vi "GlobalDrivebase.vi"() -> ()   [LabVIEW 2023]
panel:
  in  "DriveConfig":T1={"Future Proof Configs"=FALSE, "MotorOutputInverted"=0, "MotorOutputNeutralMode"=0, "MotorOutputDutyCycleNeutralDeadband"=0.0, "MotorOutputPeakForwardDutyCycle"=1.0, "MotorOutputPeakReverseDutyCycle"=-1.0, "CurrentLimitsStatorCurrentLimit"=0.0, "CurrentLimitsStatorCurrentLimitEnable"=FALSE, "CurrentLimitsSupplyCurrentLimit"=0.0, "CurrentLimitsSupplyCurrentLimitEnable"=FALSE, "CurrentLimitsSupplyCurrentThreshold"=0.0, "CurrentLimitsSupplyTimeThreshold"=0.0, "VoltageSupplyVoltageTimeConstant"=0.0, "VoltagePeakForwardVoltage"=16.0, "VoltagePeakReverseVoltage"=-16.0, "TorqueCurrentPeakForwardTorqueCurrent"=800.0, "TorqueCurrentPeakReverseTorqueCurrent"=-800.0, "TorqueCurrentTorqueNeutralDeadband"=0.0, "FeedbackFeedbackRotorOffset"=0.0, "FeedbackSensorToMechanismRatio"=1.0, "FeedbackRotorToSensorRatio"=1.0, "FeedbackFeedbackSensorSource"=0, "FeedbackFeedbackRemoteSensorID"=0, "DifferentialSensorsDifferentialSensorSource"=0, "DifferentialSensorsDifferentialTalonFXSensorID"=0, "DifferentialSensorsDifferentialRemoteSensorID"=0, "DifferentialConstantsPeakDifferentialDutyCycle"=2.0, "DifferentialConstantsPeakDifferentialVoltage"=32.0, "DifferentialConstantsPeakDifferentialTorqueCurrent"=1600.0, "OpenLoopRampsDutyCycleOpenLoopRampPeriod"=0.0, "OpenLoopRampsVoltageOpenLoopRampPeriod"=0.0, "OpenLoopRampsTorqueOpenLoopRampPeriod"=0.0, "ClosedLoopRampsDutyCycleClosedLoopRampPeriod"=0.0, "ClosedLoopRampsVoltageClosedLoopRampPeriod"=0.0, "ClosedLoopRampsTorqueClosedLoopRampPeriod"=0.0, "HardwareLimitSwitchForwardLimitType"=0, "HardwareLimitSwitchForwardLimitAutosetPositionEnable"=FALSE, "HardwareLimitSwitchForwardLimitAutosetPositionValue"=0.0, "HardwareLimitSwitchForwardLimitEnable"=TRUE, "HardwareLimitSwitchForwardLimitSource"=0, "HardwareLimitSwitchForwardLimitRemoteSensorID"=0, "HardwareLimitSwitchReverseLimitType"=0, "HardwareLimitSwitchReverseLimitAutosetPositionEnable"=FALSE, "HardwareLimitSwitchReverseLimitAutosetPositionValue"=0.0, "HardwareLimitSwitchReverseLimitEnable"=TRUE, "HardwareLimitSwitchReverseLimitSource"=0, "HardwareLimitSwitchReverseLimitRemoteSensorID"=0, "AudioBeepOnBoot"=TRUE, "AudioBeepOnConfig"=TRUE, "AudioAllowMusicDurDisable"=FALSE, "SoftwareLimitSwitchForwardSoftLimitEnable"=FALSE, "SoftwareLimitSwitchReverseSoftLimitEnable"=FALSE, "SoftwareLimitSwitchForwardSoftLimitThreshold"=0.0, "SoftwareLimitSwitchReverseSoftLimitThreshold"=0.0, "MotionMagicMotionMagicCruiseVelocity"=0.0, "MotionMagicMotionMagicAcceleration"=0.0, "MotionMagicMotionMagicJerk"=0.0, "MotionMagicMotionMagicExpo_kV"=0.0, "MotionMagicMotionMagicExpo_kA"=0.0, "CustomParamsCustomParam0"=0, "CustomParamsCustomParam1"=0, "ClosedLoopGeneralContinuousWrap"=FALSE, "Slot0kP"=0.0, "Slot0kI"=0.0, "Slot0kD"=0.0, "Slot0kS"=0.0, "Slot0kV"=0.0, "Slot0kA"=0.0, "Slot0kG"=0.0, "Slot0GravityType"=0, "Slot0StaticFeedforwardSign"=0, "Slot1kP"=0.0, "Slot1kI"=0.0, "Slot1kD"=0.0, "Slot1kS"=0.0, "Slot1kV"=0.0, "Slot1kA"=0.0, "Slot1kG"=0.0, "Slot1GravityType"=0, "Slot1StaticFeedforwardSign"=0, "Slot2kP"=0.0, "Slot2kI"=0.0, "Slot2kD"=0.0, "Slot2kS"=0.0, "Slot2kV"=0.0, "Slot2kA"=0.0, "Slot2kG"=0.0, "Slot2GravityType"=0, "Slot2StaticFeedforwardSign"=0} {"MotorOutputInverted" items=["CounterClockwise_Positive", "Clockwise_Positive"]; "MotorOutputNeutralMode" items=["Coast", "Brake"]; "FeedbackFeedbackSensorSource" items=["RotorSensor", "RemoteCANcoder", "RemotePigeon2_Yaw", "RemotePigeon2_Pitch", "RemotePigeon2_Roll", "FusedCANcoder", "SyncCANcoder"]; "DifferentialSensorsDifferentialSensorSource" items=["Disabled", "RemoteTalonFX_Diff", "RemotePigeon2_Yaw", "RemotePigeon2_Pitch", "RemotePigeon2_Roll", "RemoteCANcoder"]; "HardwareLimitSwitchForwardLimitType" items=["NormallyOpen", "NormallyClosed"]; "HardwareLimitSwitchForwardLimitSource" items=["LimitSwitchPin"=0, "RemoteTalonFX"=1, "RemoteCANifier"=2, "RemoteCANcoder"=4, "Disabled"=3]; "HardwareLimitSwitchReverseLimitType" items=["NormallyOpen", "NormallyClosed"]; "HardwareLimitSwitchReverseLimitSource" items=["LimitSwitchPin"=0, "RemoteTalonFX"=1, "RemoteCANifier"=2, "RemoteCANcoder"=4, "Disabled"=3]; "Slot0GravityType" items=["Elevator_Static", "Arm_Cosine"]; "Slot0StaticFeedforwardSign" items=["UseVelocitySign", "UseClosedLoopSign"]; "Slot1GravityType" items=["Elevator_Static", "Arm_Cosine"]; "Slot1StaticFeedforwardSign" items=["UseVelocitySign", "UseClosedLoopSign"]; "Slot2GravityType" items=["Elevator_Static", "Arm_Cosine"]; "Slot2StaticFeedforwardSign" items=["UseVelocitySign", "UseClosedLoopSign"]}
  out "SEN_Shifter_Stuck":bool[](array[boolean])
  out "SEN_Shifter_Failure":bool[](array[boolean])
  in  "SEN_Actual_Shifter_State_3":T2(ring)
  in  "SEN_Actual_Shifter_State_2":T2(ring)
  in  "SEN_Actual_Shifter_State_1":T2(ring)
  in  "SEN_Actual_Shifter_State_0":T2(ring)
  out "OUT_Heading_Locked":bool
  out "CON_Nominal_Drive_Wheel_Diameter (in)":dbl
  out "OUT_Auto-Targeting":bool
  out "SEN_Drive_Fault":bool[](array[boolean])
  out "DAT_Unlock_Azimuth":bool
  out "OUT_Azimuth_Error_3 (deg)":dbl
  out "OUT_Azimuth_Error_1 (deg)":dbl
  out "OUT_Azimuth_Error_2 (deg)":dbl
  out "OUT_Azimuth_Error_0 (deg)":dbl
  out "SEN_Drive_Raw_Velocity_2 (rpm)":dbl
  out "SEN_Drive_Raw_Velocity_3 (rpm)":dbl
  out "SEN_Drive_Raw_Velocity_1 (rpm)":dbl
  out "SEN_Drive_Raw_Velocity_0 (rpm)":dbl
  out "DAT_Auto_Targeting_Override":bool
  out "SEN_Azimuth_Position_Unwrapped_3 (deg)":dbl
  out "SEN_Azimuth_Position_Unwrapped_2 (deg)":dbl
  out "SEN_Azimuth_Position_Unwrapped_1 (deg)":dbl
  out "SEN_Azimuth_Position_Unwrapped_0 (deg)":dbl
  out "SEN_Latched_Shift_Time_3 (ms)":u32
  out "SEN_Latched_Shift_Time_2 (ms)":u32
  out "SEN_Latched_Shift_Time_1 (ms)":u32
  out "SEN_Latched_Shift_Time_0 (ms)":u32
  out "SEN_Drive_Velocity_2 (ft/s)":dbl
  out "SEN_Drive_Velocity_3 (ft/s)":dbl
  out "SEN_Drive_Velocity_1 (ft/s)":dbl
  out "SEN_Drive_Velocity_0 (ft/s)":dbl
  out "SEN_Drive_Overheat":bool[](array[boolean])
  out "SEN_Azimuth_Fault":bool[](array[boolean])
  out "SEN_Drive_Temp_2 (C)":dbl
  out "SEN_Drive_Temp_3 (C)":dbl
  out "SEN_Drive_Temp_1 (C)":dbl
  out "SEN_Drive_Temp_0 (C)":dbl
  out "SEN_Azimuth_Position_3 (deg)":dbl
  out "SEN_Azimuth_Position_2 (deg)":dbl
  out "SEN_Azimuth_Position_1 (deg)":dbl
  out "SEN_Azimuth_Position_0 (deg)":dbl
  out "OUT_Orientation Mode":enum16{"Robot-Oriented", "Field-Oriented"}(ring)
  out "OUT_Current_Driver_Profile_Setpoints":dbl[](array[numeric])
  out "OUT_Force_Low_Gear":bool
  out "OUT_High_Gear_Requested_2":bool
  out "OUT_High_Gear_Requested_1":bool
  out "OUT_High_Gear_Requested_3":bool
  out "OUT_High_Gear_Requested_0":bool
  out "OUT_Azimuth_Goal_3 (deg)":dbl
  out "OUT_Azimuth_Goal_1 (deg)":dbl
  out "OUT_Azimuth_Goal_2 (deg)":dbl
  out "OUT_Azimuth_Goal_0 (deg)":dbl
  out "OUT_Swerve_Rotation_Command":dbl
  out "OUT_Boost_Drive_Train":bool
  out "OUT_Drive_Command_3":dbl
  out "OUT_Drive_Command_1":dbl
  out "OUT_Drive_Command_2":dbl
  out "OUT_Drive_Command_0":dbl
  out "CON_Legal_Drivers":string[](array[string])
  out "DAT_New_Driver_Profile_Setpoints":dbl[](array[numeric])
  out "DAT_Apply_Driver_Profile_Setpoints":bool
  out "DAT_Starting_IMU_Reset":bool
  out "DAT_Field_Oriented_Override":bool
  out "DAT_Home_Wheels":bool
  out "DAT_Calibrate_Wheels":bool
  out "CON_Max_Robot_Rotation_Speed_(deg/s)":dbl
  out "CON_Max_Robot_Low_Gear_Speed_(ft/s)":dbl
  out "CON_Azimuth_Gear_Ratio":dbl
  out "CON_Drive_High_Gear_Ratio":dbl
  out "CON_Drive_Low_Gear_Ratio":dbl
  out "CON_Drive_Wheel_Diameter (in)":dbl
  out "CON_Robot_Width_Bumpers (in)":dbl
  out "CON_Robot_Length_Bumpers (in)":dbl
  out "CON_Robot_Minimum_Dimension (in)":dbl
  out "CON_Robot_Width (in)":dbl
  out "CON_Robot_Length (in)":dbl
  out "CON_Max_Robot_Ground_Speed_(ft/s)":dbl
  out "REF_Shifter_2":string
  out "REF_Shifter_1":string
  out "REF_Shifter_0":string
  out "REF_Shifter_3":string
  out "REF_Azimuth_3":string
  out "REF_Azimuth_2":string
  out "REF_IMU_0":string
  out "REF_Azimuth_1":string
  out "REF_Azimuth_0":string
  out "REF_Drive_3":string
  out "REF_Drive_2":string
  out "REF_Drive_1":string
  out "REF_Drive_0":string
  # "SENSORS"
  # "OUTPUTS"
  # "DRIVER STATION DATA"
  # "DEVICE REFERENCE NAMES"
  # "CONSTANTS"
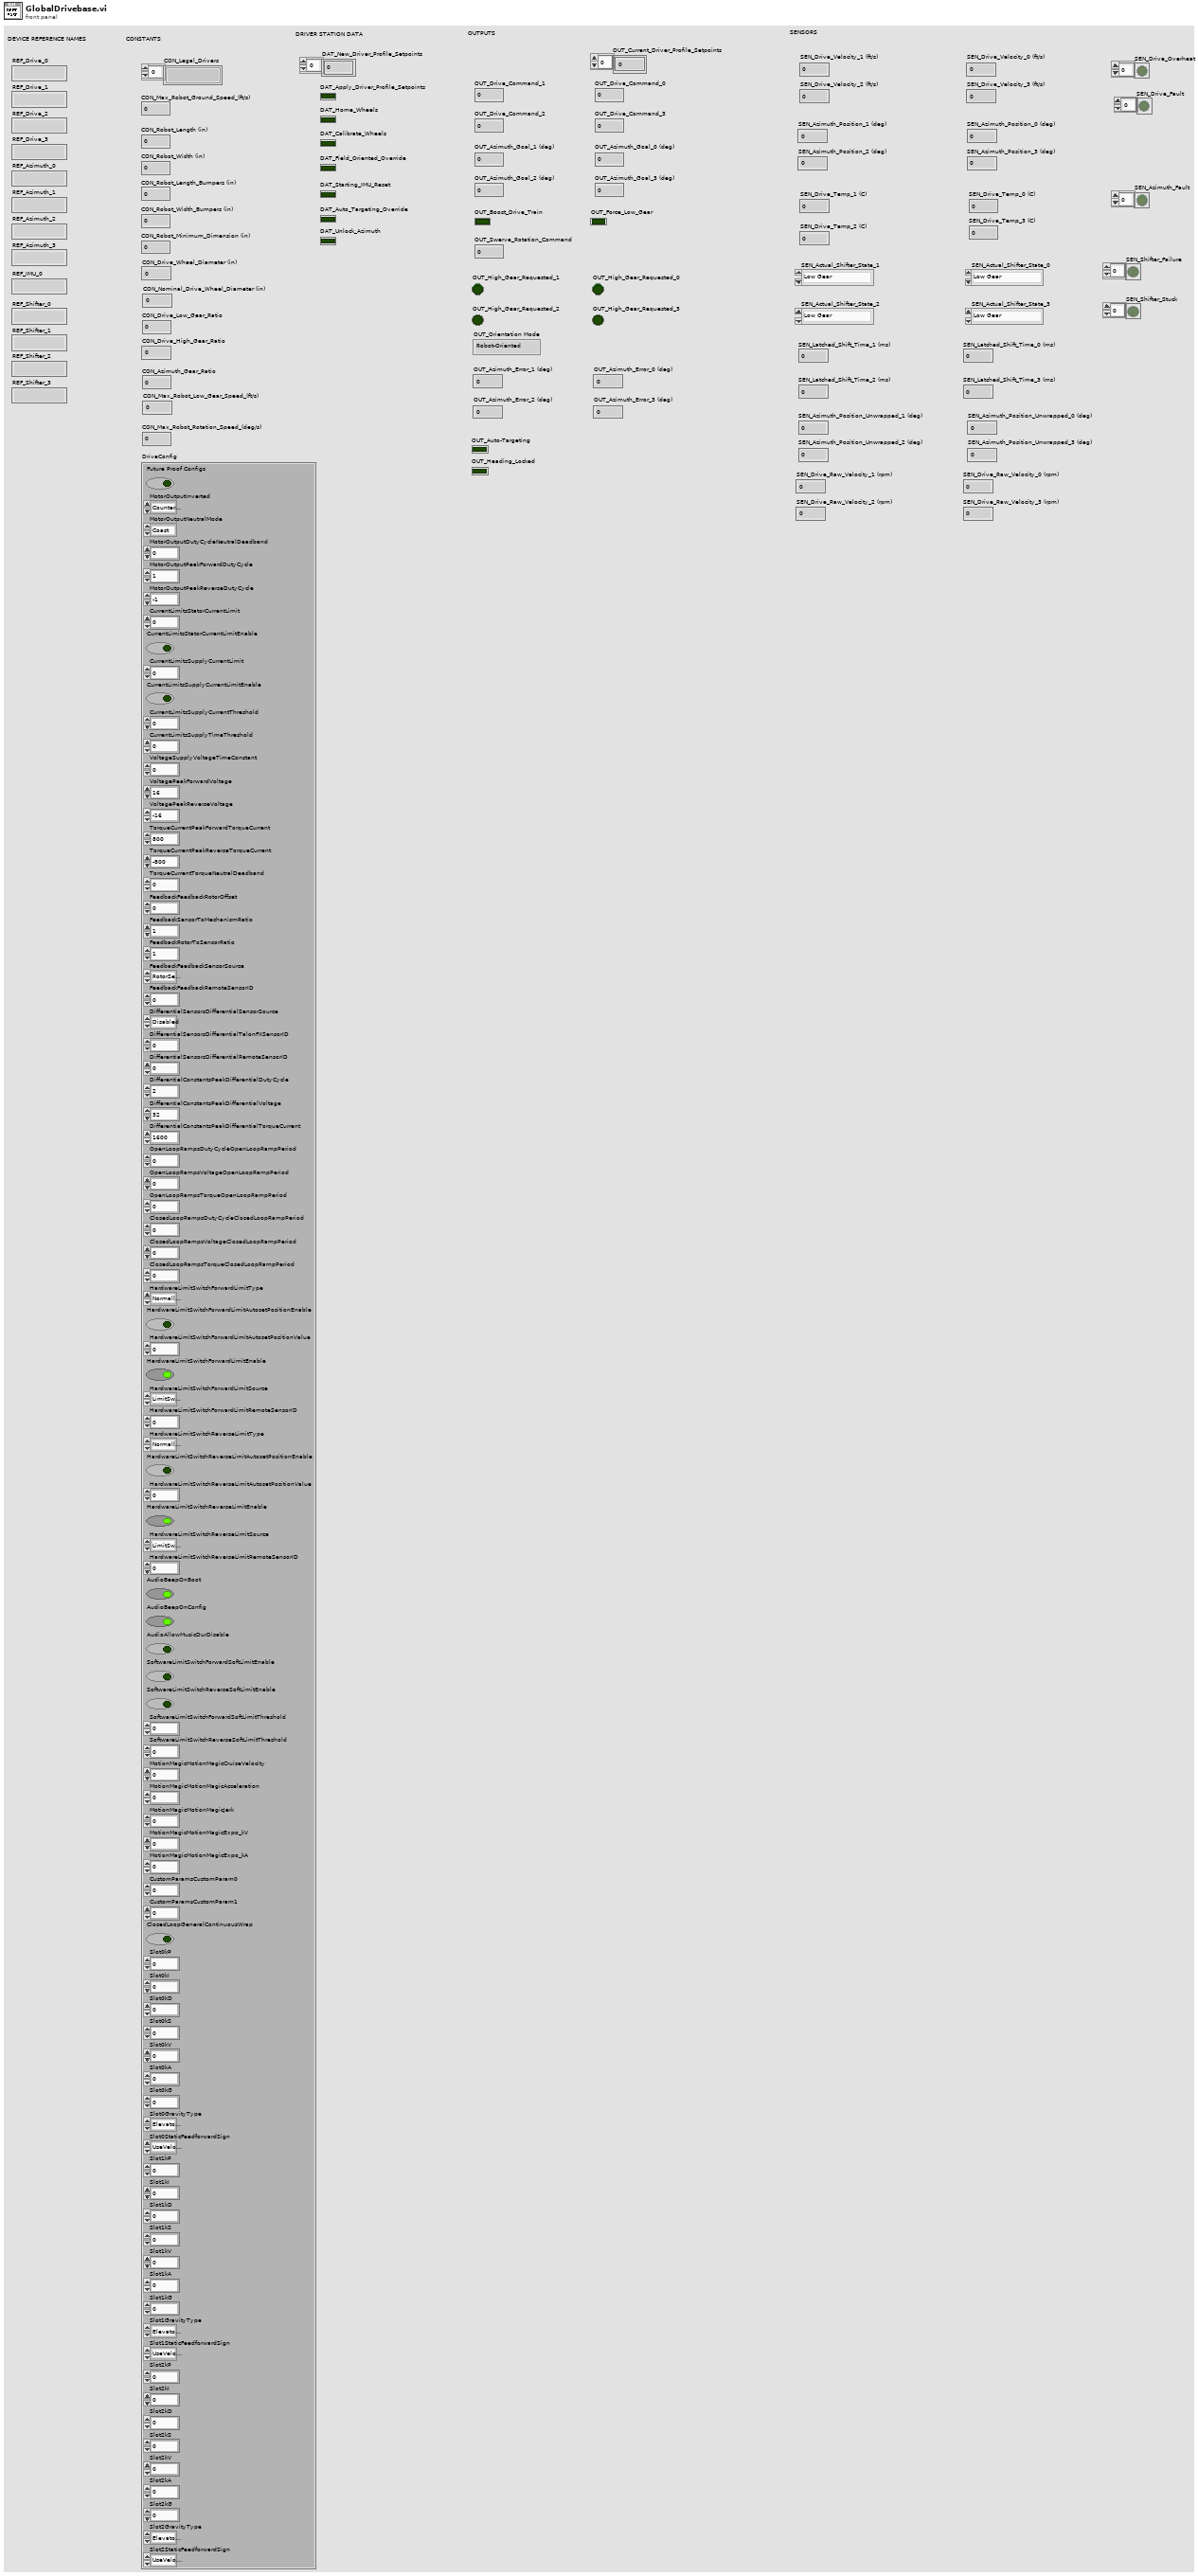
[diagram p1: front panel]
types:
  T1 = cluster{"Future Proof Configs":bool, "MotorOutputInverted":u16, "MotorOutputNeutralMode":u16, "MotorOutputDutyCycleNeutralDeadband":dbl, "MotorOutputPeakForwardDutyCycle":dbl, "MotorOutputPeakReverseDutyCycle":dbl, "CurrentLimitsStatorCurrentLimit":dbl, "CurrentLimitsStatorCurrentLimitEnable":bool, "CurrentLimitsSupplyCurrentLimit":dbl, "CurrentLimitsSupplyCurrentLimitEnable":bool, "CurrentLimitsSupplyCurrentThreshold":dbl, "CurrentLimitsSupplyTimeThreshold":dbl, "VoltageSupplyVoltageTimeConstant":dbl, "VoltagePeakForwardVoltage":dbl, "VoltagePeakReverseVoltage":dbl, "TorqueCurrentPeakForwardTorqueCurrent":dbl, "TorqueCurrentPeakReverseTorqueCurrent":dbl, "TorqueCurrentTorqueNeutralDeadband":dbl, "FeedbackFeedbackRotorOffset":dbl, "FeedbackSensorToMechanismRatio":dbl, "FeedbackRotorToSensorRatio":dbl, "FeedbackFeedbackSensorSource":u16, "FeedbackFeedbackRemoteSensorID":i16, "DifferentialSensorsDifferentialSensorSource":u16, "DifferentialSensorsDifferentialTalonFXSensorID":i16, "DifferentialSensorsDifferentialRemoteSensorID":i16, "DifferentialConstantsPeakDifferentialDutyCycle":dbl, "DifferentialConstantsPeakDifferentialVoltage":dbl, "DifferentialConstantsPeakDifferentialTorqueCurrent":dbl, "OpenLoopRampsDutyCycleOpenLoopRampPeriod":dbl, "OpenLoopRampsVoltageOpenLoopRampPeriod":dbl, "OpenLoopRampsTorqueOpenLoopRampPeriod":dbl, "ClosedLoopRampsDutyCycleClosedLoopRampPeriod":dbl, "ClosedLoopRampsVoltageClosedLoopRampPeriod":dbl, "ClosedLoopRampsTorqueClosedLoopRampPeriod":dbl, "HardwareLimitSwitchForwardLimitType":u16, "HardwareLimitSwitchForwardLimitAutosetPositionEnable":bool, "HardwareLimitSwitchForwardLimitAutosetPositionValue":dbl, "HardwareLimitSwitchForwardLimitEnable":bool, "HardwareLimitSwitchForwardLimitSource":u16, "HardwareLimitSwitchForwardLimitRemoteSensorID":i16, "HardwareLimitSwitchReverseLimitType":u16, "HardwareLimitSwitchReverseLimitAutosetPositionEnable":bool, "HardwareLimitSwitchReverseLimitAutosetPositionValue":dbl, "HardwareLimitSwitchReverseLimitEnable":bool, "HardwareLimitSwitchReverseLimitSource":u16, "HardwareLimitSwitchReverseLimitRemoteSensorID":i16, "AudioBeepOnBoot":bool, "AudioBeepOnConfig":bool, "AudioAllowMusicDurDisable":bool, "SoftwareLimitSwitchForwardSoftLimitEnable":bool, "SoftwareLimitSwitchReverseSoftLimitEnable":bool, "SoftwareLimitSwitchForwardSoftLimitThreshold":dbl, "SoftwareLimitSwitchReverseSoftLimitThreshold":dbl, "MotionMagicMotionMagicCruiseVelocity":dbl, "MotionMagicMotionMagicAcceleration":dbl, "MotionMagicMotionMagicJerk":dbl, "MotionMagicMotionMagicExpo_kV":dbl, "MotionMagicMotionMagicExpo_kA":dbl, "CustomParamsCustomParam0":i16, "CustomParamsCustomParam1":i16, "ClosedLoopGeneralContinuousWrap":bool, "Slot0kP":dbl, "Slot0kI":dbl, "Slot0kD":dbl, "Slot0kS":dbl, "Slot0kV":dbl, "Slot0kA":dbl, "Slot0kG":dbl, "Slot0GravityType":u16, "Slot0StaticFeedforwardSign":u16, "Slot1kP":dbl, "Slot1kI":dbl, "Slot1kD":dbl, "Slot1kS":dbl, "Slot1kV":dbl, "Slot1kA":dbl, "Slot1kG":dbl, "Slot1GravityType":u16, "Slot1StaticFeedforwardSign":u16, "Slot2kP":dbl, "Slot2kI":dbl, "Slot2kD":dbl, "Slot2kS":dbl, "Slot2kV":dbl, "Slot2kA":dbl, "Slot2kG":dbl, "Slot2GravityType":u16, "Slot2StaticFeedforwardSign":u16}
  T2 = enum16{"Low Gear", "High Gear", "Transiting", "Unknown", "Force Low Gear"}
diagram:
